vi "Troughput_SubVI.vi"(8 "Show File in Explorer":bool=TRUE, 10 "path":path, 11 "URL":string) -> (0 "error out":errorcluster, 1 "size (in bytes)":i64, 3 "Indicator":bool)   [LabVIEW 2017]
uses:
  Global Stop Variable.vi
  <vilib>/httpClient/LabVIEWHTTPClient.lvlib
panel:
  out "File name":string
  out "headers":string
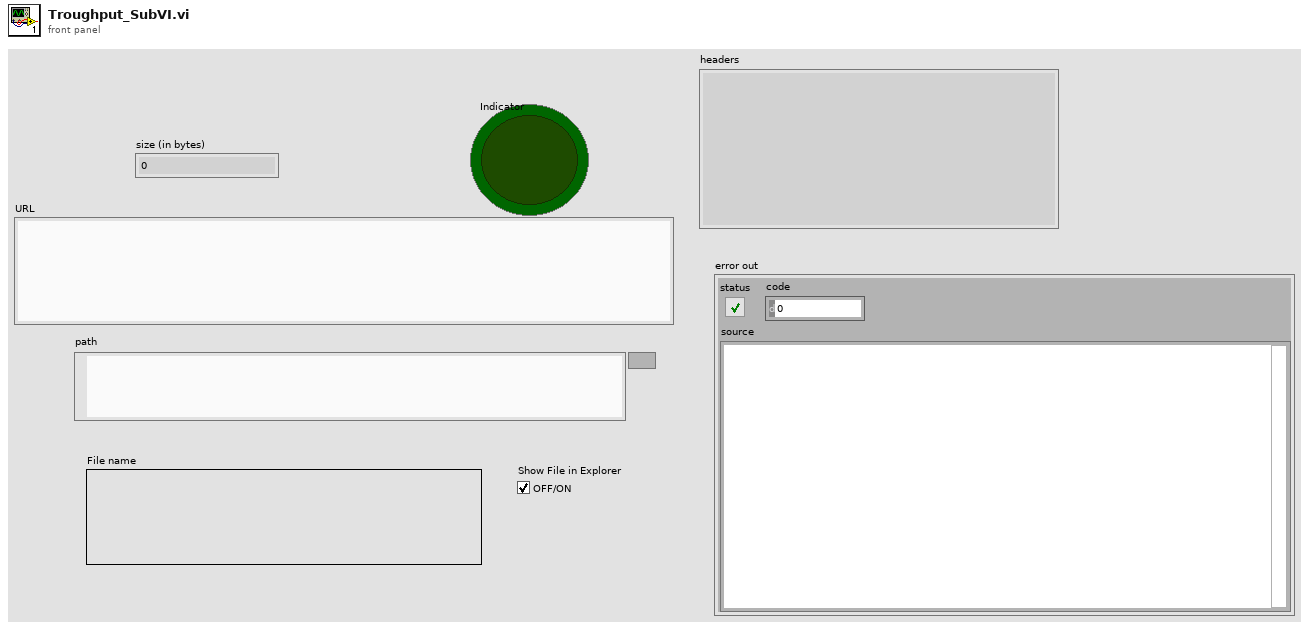
[diagram p1: front panel]
types:
  T1 = typedef "LabVIEWHTTPClient.lvlib/ClientHandle.ctl" = refnum<k1>
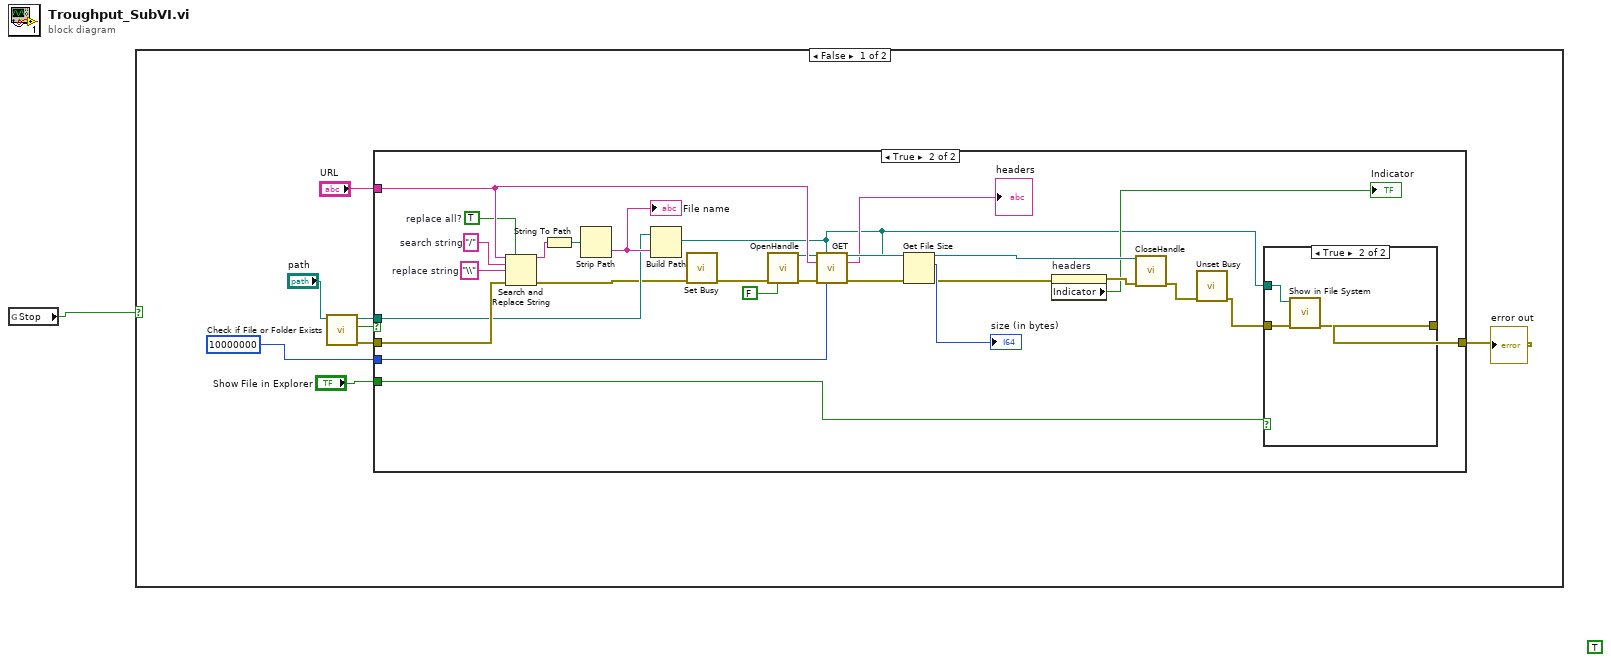
[diagram p0: block diagram]
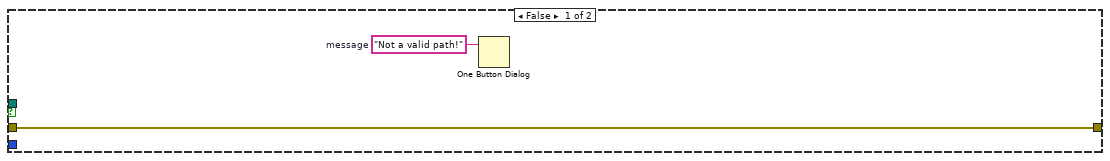
[diagram p2: hidden frame]
diagram:
  (unwired) TRUE
  n1 = global read "Global Stop Variable.vi" "Stop"() -> (w1:bool)
  n2 = case shown="False" w1 {
    frame False {
      n3 = call <vilib>:"Check if File or Folder Exists.vi"("path"="path") -> ("error out"=w9:errorcluster, "file or folder exists?"=w2:bool, "dup path"=w8:path)  [unwired: 8 in]
      n4 = case shown="True" w2 {
        tunnel: "URL" -> [_ w38]
        tunnel: w9 -> [w11 w31]
        tunnel: w8 -> [_ w30]
        tunnel: [w11 w26] -> w7
        tunnel: "Show File in Explorer" -> [_ w25]
        tunnel: 10000000 ("timeout (10000)") -> [_ w24]
        frame False {
          w10 = "Not a valid path!"  # message
          n5 = One Button Dialog(message=w10) -> ()  [unwired: 1 in, 1 out]
        }
        frame True {
          w35 = TRUE  # replace all?
          w36 = "\\"  # replace string
          w37 = "/"  # search string
          n6 = Search and Replace String(replace all?=w35, input string=w38, search string=w37, replace string=w36, error in=w31) -> (result string=w34:string, error out=w21:errorcluster)  [unwired: 3 in, 2 out]
          n7 = String To Path(string=w34) -> (path=w33:path)
          n8 = Strip Path(path=w33) -> (name=w32:string)  [unwired: 1 out]
          "File name" <- w32
          n9 = Build Path(base path=w30, name or relative path=w32) -> (appended path=w15:path)
          n10 = call <vilib>:"Set Busy.vi"("error in (no error)"=w21) -> ("error out"=w20:errorcluster)  [unwired: 9 in, 1 out]
          n11 = call <vilib>:"OpenHandle.vi"("error in (no error)"=w20, "verify server(true)"=FALSE) -> ("client handle out"=w27:T1, "error out"=w28:errorcluster)  [unwired: 12 in]
          n12 = call <vilib>:"GET.vi"("client handle"=w27, "output file"=w15, "url"=w38, "error in (no error)"=w28, "timeout (10000)"=w24) -> ("client handle out"=w29:T1, "headers"=→"headers":string, "error out"=w14:errorcluster)  [unwired: 7 in, 1 out]
          n13 = Get File Size(file=w15, error in=w14) -> (size (in bytes)=→"size (in bytes)":i64, 0:w13:errorcluster)  [unwired: 1 out]
          n14 = property on="headers" class="Str"(error in=w13) -> (error out=w18:errorcluster, "Indicator"=→"Indicator":bool)  [unwired: 1 in, 1 out]
          n15 = call <vilib>:"CloseHandle.vi"("client handle"=w29, "error in (no error)"=w18) -> ("error out"=w23:errorcluster)  [unwired: 13 in]
          n16 = call <vilib>:"Unset Busy.vi"("error in (no error)"=w23) -> ("error out"=w22:errorcluster)  [unwired: 10 in]
          n17 = case shown="True" w25 {
            tunnel: w15 -> [_ w40]
            tunnel: w22 -> [w39 w42]
            tunnel: [w39 w41] -> w26
            frame False {
            }
            frame True {
              n18 = call <vilib>:"Show in File System.vi"("error in (no error)"=w42, "file or directory path"=w40) -> ("error out"=w41:errorcluster)  [unwired: 9 in]
            }
          }
        }
      }
      "error out" <- w7
    }
    frame True {
    }
  }
